vi "PhotonPipelineMetadata_GetAll.vi"(11 "PhotonPipelineMetadata":T1={"CaptureTimestampMicros"=-1, "PublishTimestampMicros"=-1, "SequenceID"=-1, "TimeSinceLastPong"=9999999999}) -> (0 "TimeSinceLastPong":i64, 1 "SequenceID":i64, 2 "PublishTimestampMicros":i64, 3 "CaptureTimestampMicros":i64)   [LabVIEW 2019, in "PhotonVisionLib.lvlib"]
doc: "Returns individual elements of PipelineMetadata cluster\n\nInputs:\n - PipelineMetadata -- Parsed PipelineMetadata cluster.\n\nOutputs:\n - CaptureTimestampMicros -- Image capture timestamp, in microseconds\n - PublishTimestampMicros -- NT publish timestamp, in microseconds\n - SequenceID -- Mirror of the heartbeat entry -- monotonically increasing\n - TimeSinceLastPong -- Time from last Time Sync Pong received and the construction of this metadata, in uS"
uses:
  PhotonVisionLib.lvlib
  TypeDef/PhotonPipelineMetadataType.ctl
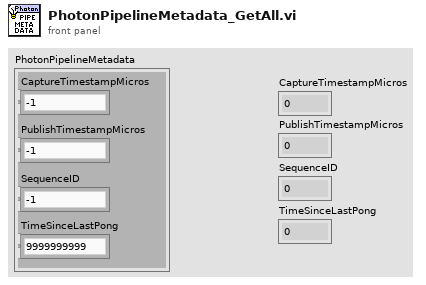
[diagram p1: front panel]
types:
  T1 = typedef "PhotonVisionLib.lvlib/PhotonPipelineMetadataType.ctl" = cluster{"CaptureTimestampMicros":i64, "PublishTimestampMicros":i64, "SequenceID":i64, "TimeSinceLastPong":i64}
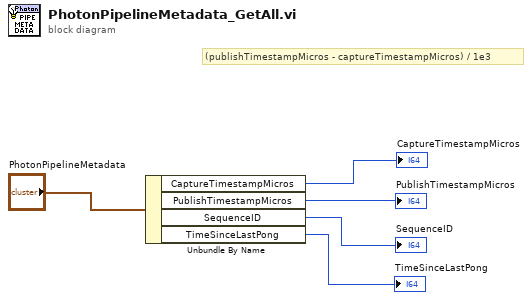
[diagram p0: block diagram]
diagram:
  # "(publishTimestampMicros - captureTimestampMicros) / 1e3"
  n1 = Unbundle By Name("PhotonPipelineMetadata") -> ("CaptureTimestampMicros"=→"CaptureTimestampMicros":i64, "PublishTimestampMicros"=→"PublishTimestampMicros":i64, "SequenceID"=→"SequenceID":i64, "TimeSinceLastPong"=→"TimeSinceLastPong":i64)
